vi "Guardian Died Recheck.vi"(8 "error in (no error)":errorcluster, 10 "ID":string, 11 "Guardian in":refnum<class "Guardian.lvclass">) -> (0 "error out":errorcluster, 3 "Guardian out":refnum<class "Guardian.lvclass">)   [LabVIEW 2026, in "TALOS.lvlib" / "Guardian.lvlib" / "Guardian.lvclass"]
doc: "This VI gets scheduled to be run whenever a Guardian is found to be not updating its Guardian_Health ASV: if the Guardian is found alive, nothing is done, while if it is really found dead, ABORT is raised."
uses:
  Guardian.lvclass
  C:/LabVIEW Code/TALOS/talos/Ancestor/Ancestor/Ancestor.lvclass
  Guardian.lvclass/Guardian.ctl
  Ancestor/Ancestor/Ancestor.lvclass/Ancestor.ctl
  b6742f5d-21ec-4deb-8824-cf1d71f74dd0.vi
  Ancestor/Ancestor/Write Distr uS Map ref.vi
  Write Guardian List.vi
  Read Bearer.vi
  Ancestor/Ancestor/Read Distr uS Map ref.vi
  Read Guardian List.vi
  FGV/Error Memory/Get Error Description.vi
  Support VIs/Get PC name.vi
  Support VIs/Get Class Name.vi
  <vilib>/Utility/error.llb/Clear Errors.vi
  FGV/Error Memory/Error Memory Core.vi
  <vilib>/AdvancedString/Delimited String to 1D String Array.vi
  <vilib>/AdvancedString/Delimited String to 1D String Array (string).vi
  Support VIs/Circus Root Path.vi
  FGV/Error Memory/Error Crt Lvl checker.vi
  FGV/Error Memory/Error Memory Core.vi/40c8088d-b597-4017-91af-faa98e00292e.vi
  FGV/Error Memory/Error Memory Core.vi/d4a3ab98-063c-4e44-b43d-fbdcfe6c2be2.vi
  Support VIs/Global Memory.vi
  <vilib>/Utility/LVClass/Get LV Class Name.vi
  Support VIs/Is in Packed Library.vi
  Support VIs/TALOS Root path.vi
  Support VIs/Read CSV worksheet.vi
  Support VIs/Global Constants.vi
  <vilib>/Utility/error.llb/General Error Handler.vi
  Classes/Guardian List/Guardian List.lvclass
  Classes/Distributed uService Map/Distributed uService Map.lvclass
  <vilib>/Comparison/Less/Less Functor/Less Functor.lvclass
  Ancestor/Ancestor/Ancestor.lvclass
  <vilib>/Comparison/Equal/Equal Functor/Equal Functor.lvclass
  TALOS.lvlib
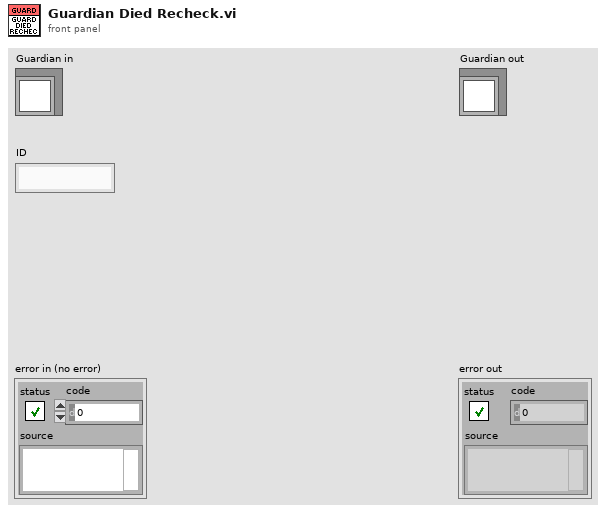
[diagram p1: front panel]
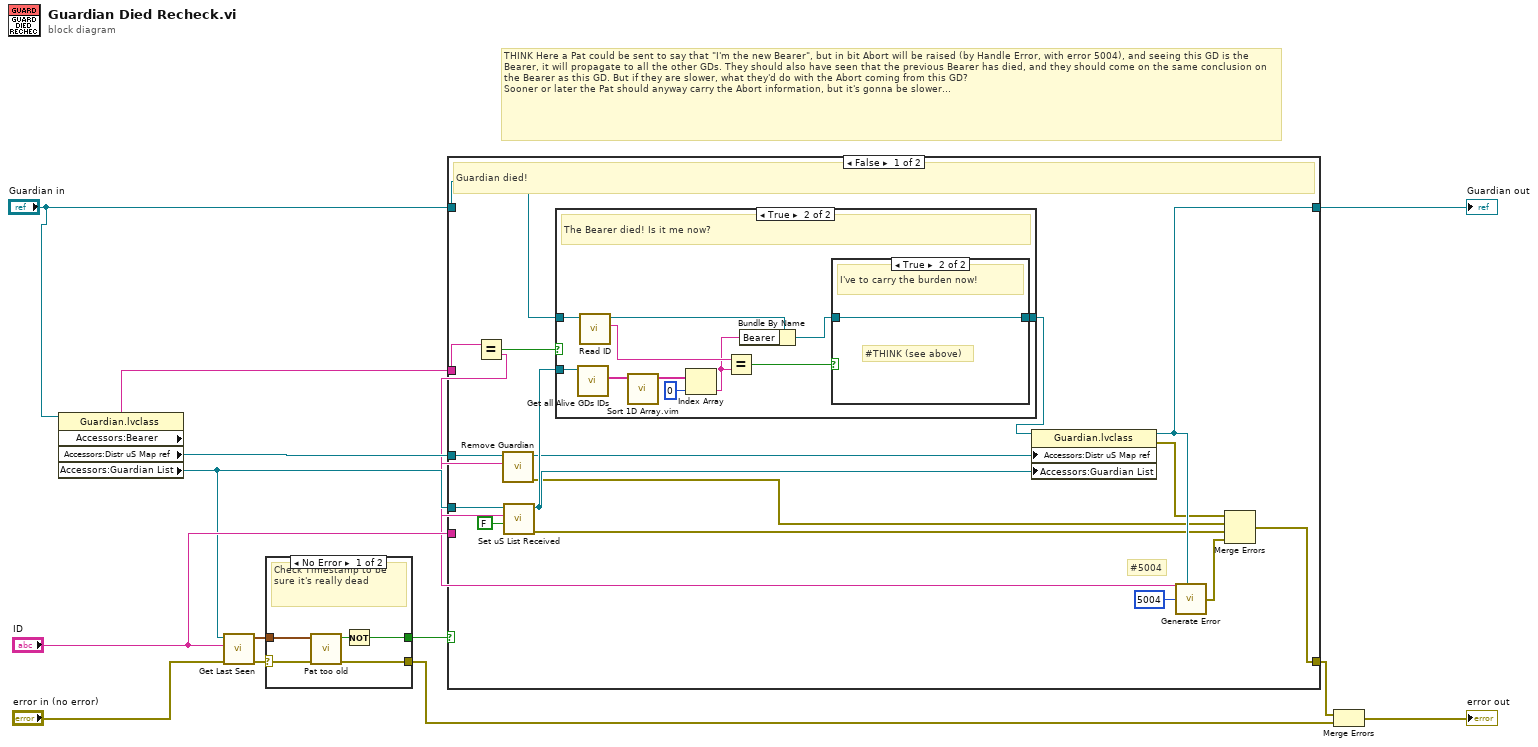
[diagram p0: block diagram]
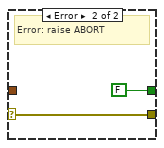
[diagram p2: hidden frame]
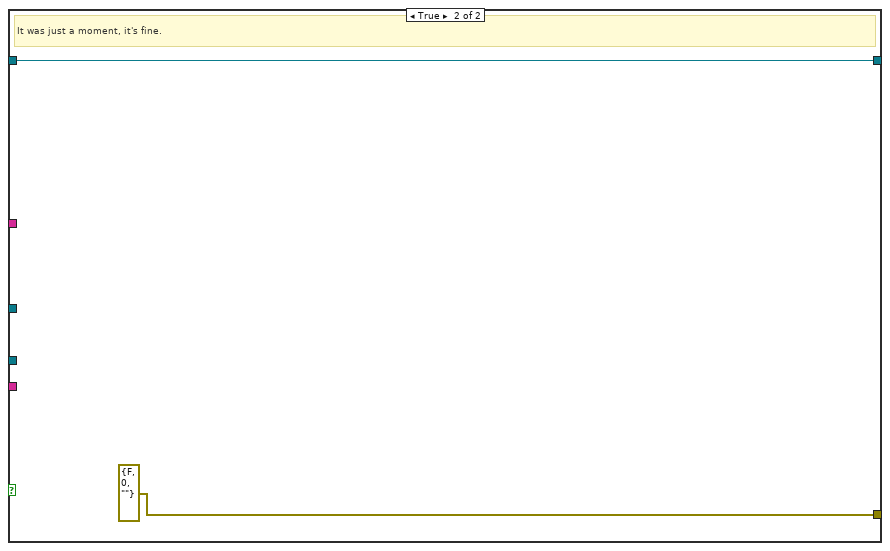
[diagram p5: hidden frame]
diagram:
  # "THINK Here a Pat could be sent to say that \"I'm the new Bearer\", but in bit Abort will be raised (by Handle Error, with error 5004), and seeing this GD is the Bearer, it will propagate to all the other GDs. They should also have seen that the previous Bearer has died, and they should come on the same conclusion on the Bearer as this GD. But if they are slower, what they'd do with the Abort coming from this GD? \nSooner or later the Pat should anyway carry the Abort information, but it's gonna be slower..."
  n1 = property class="Guardian.lvclass"(reference="Guardian in") -> ("Accessors:Bearer"=w3:string, "Accessors:Distr uS Map ref"=w2:refnum<data-value>, "Accessors:Guardian List"=w1:refnum<class "Guardian List.lvclass">)  [unwired: 1 in, 2 out]
  n2 = call-dynamic "Get Last Seen.vi"("error in (no error)"="error in (no error)", "ID"="ID", "Guardian List in"=w1) -> ("error out"=w8:errorcluster, "Last Poke"=w9:timestamp)  [unwired: 6 in, 1 out]
  n3 = case shown="No Error" w8 {
    selector: w8 -> [w15 w19]
    tunnel: w9 -> [w18 _]
    tunnel: [w16 FALSE] -> w11
    tunnel: [w14 w19] -> w7
    frame No Error {
      # "Check Timestamp to be sure it's really dead"
      n4 = call "Pat too old.vi"("error in (no error)"=w15, "Last Seen"=w18) -> ("error out"=w14:errorcluster, "Too old?"=w17:bool)  [unwired: 8 in]
      n5 = Not(x=w17) -> (.not. x?=w16:bool)
    }
    frame Error {
      # "Error: raise ABORT"
    }
  }
  n6 = case shown="False" w11 {
    tunnel: [w28 errorcluster {"status"=FALSE, "code"=0, "source"=""} ("error out")] -> w12
    tunnel: "Guardian in" -> [w30 w52]
    tunnel: w1 -> [w36 _]
    tunnel: "ID" -> [w33 _]
    tunnel: [w26 w52] -> w4
    tunnel: w2 -> [w34 _]
    tunnel: w3 -> [w29 _]
    frame False {
      # "#5004"
      # "Guardian died!"
      n7 = Equal?(x=w29, y=w33) -> (x = y?=w32:bool)
      n8 = call "Remove Guardian.vi"("Guardian ID"=w33, "Distr uS Map ref in"=w34) -> ("error out"=w23:errorcluster, "Distr uS Map ref out"=w22:refnum<data-value>)  [unwired: 8 in]
      n9 = call-dynamic "Set uS List Received.vi"("uS List Received"=FALSE, "ID"=w33, "Guardian List in"=w36) -> ("error out"=w21:errorcluster, "Guardian List out"=w31:refnum<class "Guardian List.lvclass">)  [unwired: 7 in]
      n10 = case shown="True" w32 {
        tunnel: w31 -> [_ w49]
        tunnel: w30 -> [w38 w47]
        tunnel: [w38 w41] -> w24
        frame False {
          # "The dead GD was not the Bearer, all good."
        }
        frame True {
          # "The Bearer died! Is it me now?"
          n11 = call-dynamic "Get all Alive GDs IDs.vi"("Guardian List in"=w49) -> ("Alive GDs IDs"=w39:string[])  [unwired: 8 in, 2 out]
          n12 = call "Read ID.vi"("Ancestor in"=w47) -> ("ID"=w44:string, "Ancestor out"=w45:refnum<class "Guardian.lvclass">)  [unwired: 8 in, 1 out]
          n13 = call "Sort 1D Array.vim"("unsorted array"=w39) -> ("sorted array"=w40:string[])  [unwired: 10 in]
          n14 = Index Array(array=w40, index=0) -> (element=w43:string)
          n15 = Equal?(x=w44, y=w43) -> (x = y?=w46:bool)
          n16 = Bundle By Name(cluster=w45, "Bearer"=w43) -> (w42:refnum<class "Guardian.lvclass">)
          n17 = case shown="True" w46 {
            tunnel: w42 -> [w50 w51]
            tunnel: [w50 w51] -> w41
            frame False {
              # "No (do nothing)"
            }
            frame True {
              # "#THINK (see above)"
              # "I've to carry the burden now!"
            }
          }
        }
      }
      n18 = property class="Guardian.lvclass"(reference=w24, "Accessors:Distr uS Map ref"=w22, "Accessors:Guardian List"=w31) -> (reference out=w26:refnum<class "Guardian.lvclass">, error out=w25:errorcluster)  [unwired: 1 in]
      n19 = call "Generate Error.vi"("Optional String"=w33, "Class"=w26, "Error Code"=5004) -> ("error out"=w27:errorcluster)  [unwired: 4 in]
      n20 = Merge Errors(w25, w23, w21, w27) -> (w28:errorcluster)
    }
    frame True {
      # "It was just a moment, it's fine."
    }
  }
  "Guardian out" <- w4
  n21 = Merge Errors(w12, w7) -> (→"error out":errorcluster)
